vi "Bertta_v02.vi"() -> ()   [LabVIEW 2015]
uses:
  BERTTA.dll
panel:
  in  "col":i32=3
  out "values":dbl[](array[numeric])
  out "Mettler":dynamicdata(graph)
  in  "?":T1(tab)
  out "rc":i32
  in  "Kd":dbl
  in  "Ki":dbl
  in  "Kp":dbl=2.0
  out "PID output":dbl
  in  "Temp setpoint":dbl=20.0
  in  "Device port":dbl=1.0
  out "Debug msg":dbl
  out "Temp Lauda":dbl
  out "Timestep":i32
  in  "Device port":i32=2
  out "Weight":dbl
  out "Weight":dbl
  in  "Device port":i32=6
  out "Lauda":dynamicdata(graph)
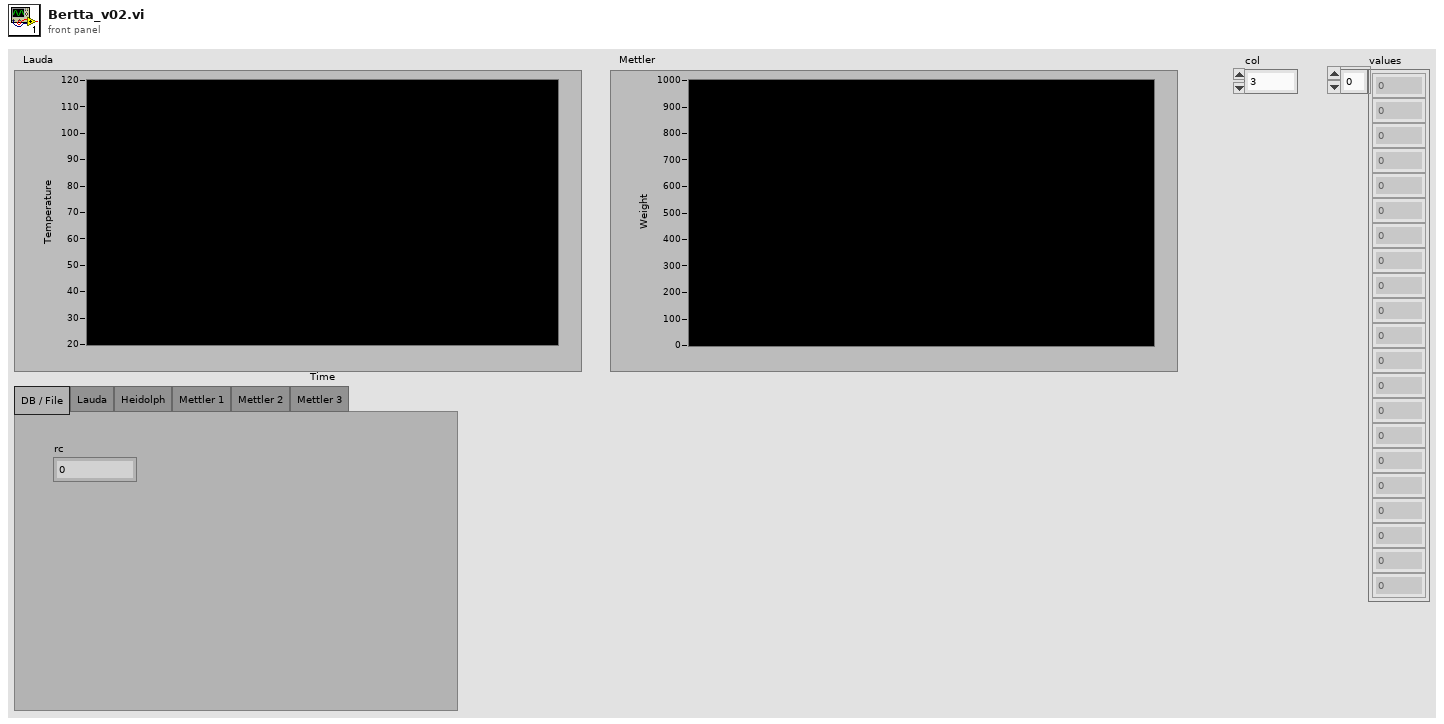
[diagram p1: front panel]
types:
  T1 = enum32{"DB / File", "Lauda", "Heidolph", "Mettler 1", "Mettler 2", "Mettler 3"}
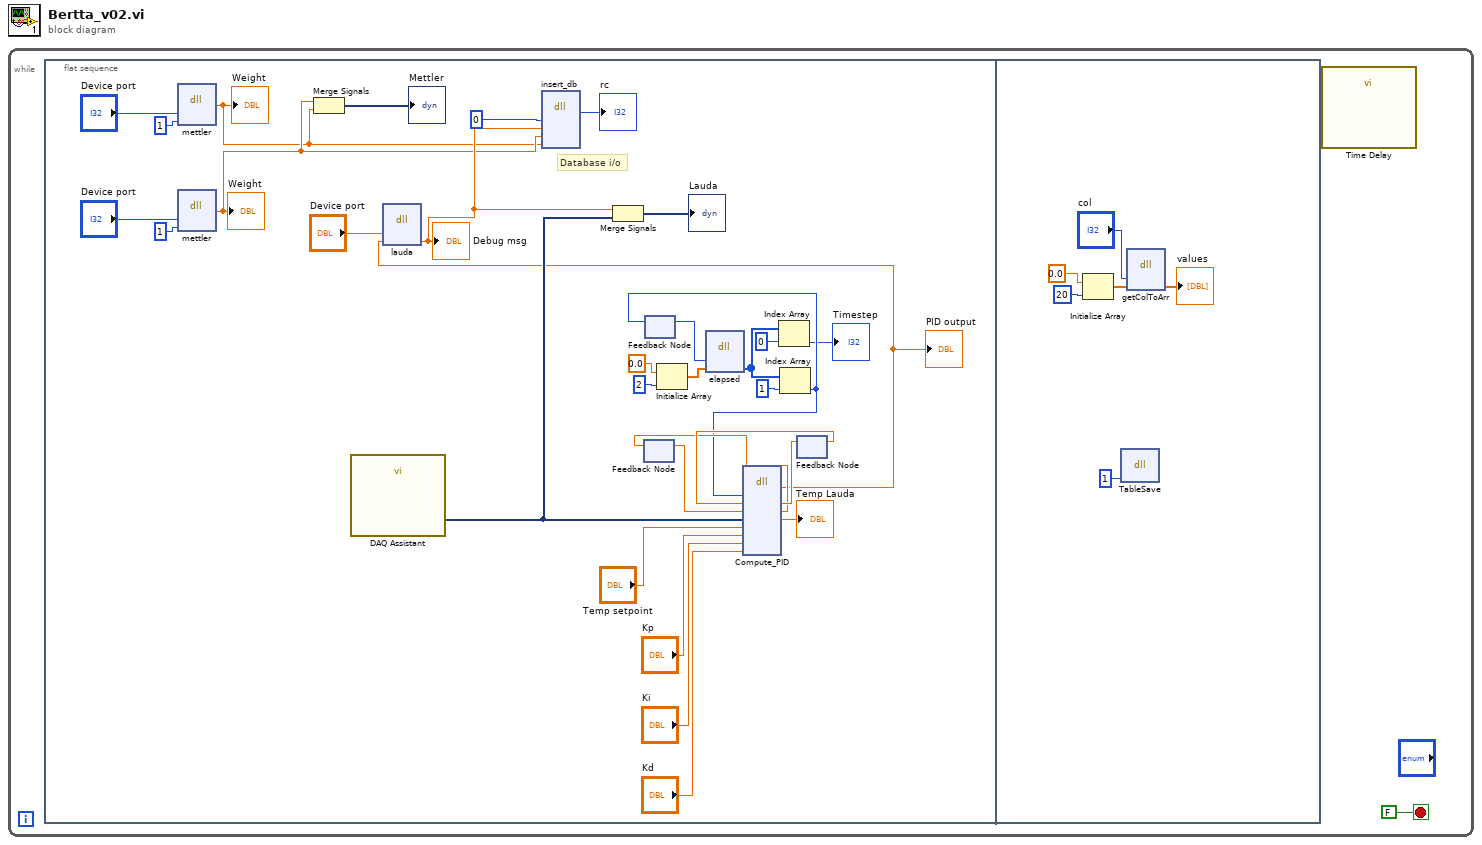
[diagram p0: block diagram]
diagram:
  n1 = while {
    stop <- FALSE stop-if-true
    n2 = flat-sequence {
      frame #0 {
        # "Database i/o"
        n3 = dll-call lib="C:/Users/xlaraser/Documents/Visual Studio 2017/Projects/Bertta/BERTTA/Debug/BERTTA.dll" fn="mettler"("port"="Device port", "msg"=1) -> ("return type"=w12:dbl)  [unwired: 5 in, 2 out]
        "Weight" <- w12
        n4 = dll-call lib="C:/Users/xlaraser/Documents/Visual Studio 2017/Projects/Bertta/BERTTA/Debug/BERTTA.dll" fn="mettler"("port"="Device port", "msg"=1) -> ("return type"=w13:dbl)  [unwired: 5 in, 2 out]
        "Weight" <- w13
        n5 = Merge Signals(w13, w12) -> (→"Mettler":dynamicdata)
        n6 = call "DAQ Assistant"() -> ("data"=w24:dynamicdata)  [unwired: 17 in, 2 out]
        n7 = feedback #1() -> (w28:dbl)  [unwired: 1 in]
        n8 = feedback #2() -> (w9:i32)  [unwired: 1 in]
        n9 = Initialize Array(0.0 ("element"), 2 ("dimension size")) -> (w7:dbl[])
        n10 = dll-call lib="C:/Users/xlaraser/Documents/Visual Studio 2017/Projects/Bertta/BERTTA/Debug/BERTTA.dll" fn="elapsed"("last_time"=w9, "params"=w7) -> ("params"=w3:i32[])  [unwired: 5 in, 2 out]
        n11 = Index Array(array=w3, index=0) -> (element=→"Timestep":i32)
        n12 = Index Array(array=w3, index=1) -> (element=w5:i32)
        n13 = feedback-in #2(w5) -> ()
        n14 = feedback #3() -> (w30:dbl)  [unwired: 1 in]
        n15 = dll-call lib="C:/Users/xlaraser/Documents/Visual Studio 2017/Projects/Bertta/BERTTA/Debug/BERTTA.dll" fn="Compute_PID"("timeChange"=w5, "errSum"=w30, "lastErr"=w28, "Input"=w24, "Setpoint"="Temp setpoint", "kp"="Kp", "ki"="Ki", "kd"="Kd") -> ("return type"=w22:dbl, "errSum"=w31:dbl, "lastErr"=w29:dbl, "Input"=→"Temp Lauda":dbl)  [unwired: 8 in, 2 out]
        "PID output" <- w22
        n16 = dll-call lib="C:/Users/xlaraser/Documents/Visual Studio 2017/Projects/Bertta/BERTTA/Debug/BERTTA.dll" fn="lauda"("port"="Device port", "set_temp"=w22) -> ("set_temp"=w26:dbl)  [unwired: 5 in, 2 out]
        "Debug msg" <- w26
        n17 = dll-call lib="C:/Users/xlaraser/Documents/Visual Studio 2017/Projects/Bertta/BERTTA/Debug/BERTTA.dll" fn="insert_db"("heidolph"=0, "lauda"=w26, "mettler1"=w13, "mettler2"=w12) -> ("return type"=→"rc":i32)  [unwired: 7 in, 2 out]
        n18 = Merge Signals(w26, w24) -> (→"Lauda":dynamicdata)
        n19 = feedback-in #1(w29) -> ()
        n20 = feedback-in #3(w31) -> ()
      }
      frame #1 {
        n21 = Initialize Array(0.0 ("element"), 20 ("dimension size")) -> (w35:dbl[])
        n22 = dll-call lib="C:/Users/xlaraser/Documents/Visual Studio 2017/Projects/Bertta/BERTTA/Debug/BERTTA.dll" fn="TableSave"("exec"=1) -> ()  [unwired: 5 in, 2 out]
        n23 = dll-call lib="C:/Users/xlaraser/Documents/Visual Studio 2017/Projects/Bertta/BERTTA/Debug/BERTTA.dll" fn="getColToArr"("col"="col", "values"=w35) -> ("values"=→"values":dbl[])  [unwired: 5 in, 2 out]
      }
    }
    n24 = call "Time Delay"() -> ()  [unwired: 11 in, 1 out]
  }
